vi "Publish To Topic.vi"(8 "error in (no error)":errorcluster, 9 "Message":string, 10 "Subject(\"\")":string, 11 "Topic in":refnum<class "Topic.lvclass">) -> (0 "error out":errorcluster, 3 "Topic out":refnum<class "Topic.lvclass">)   [LabVIEW 2018, in "NI_AWS_SNS.lvlib" / "Topic.lvclass"]
doc: "Publish a message to a SNS topic"
uses:
  Topic.lvclass
  C:/labview-projects/aws-toolkit/source/Core/ARN/ARN.lvclass
  C:/labview-projects/aws-toolkit/source/Core/HTTP Request/HTTP Request.lvclass
  Core/HTTP Request/Request Options.ctl
  Core/HTTP Request/Name Value Pair.ctl
  Core/HTTP Request/Region handling.ctl
  Core/HTTP Request/URL formatting.ctl
  Core/ARN/ARN.lvclass/ARN.ctl
  Core/ARN/Read ARN.vi
  Core/HTTP Request/HTTP Request.lvclass
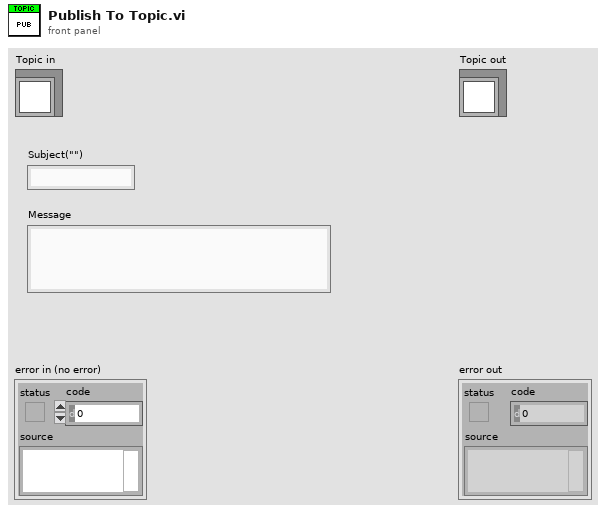
[diagram p1: front panel]
types:
  T1 = typedef "NI_AWS_Core.lvlib/HTTP Request.lvclass/Name Value Pair.ctl" = cluster{"name":string, "value":string}
  T2 = typedef "NI_AWS_Core.lvlib/HTTP Request.lvclass/Request Options.ctl" = cluster{"request headers":T1[], "request parameters":T1[], "request body":string, "region handling":T3, "URL formatting":T4}
  T3 = typedef "NI_AWS_Core.lvlib/HTTP Request.lvclass/Region handling.ctl" = enum16{"use region everywhere", "use region (authentication only)", "use region (URL only)", "ignore region everwhere"}
  T4 = typedef "NI_AWS_Core.lvlib/HTTP Request.lvclass/URL formatting.ctl" = enum16{"region-", "region."}
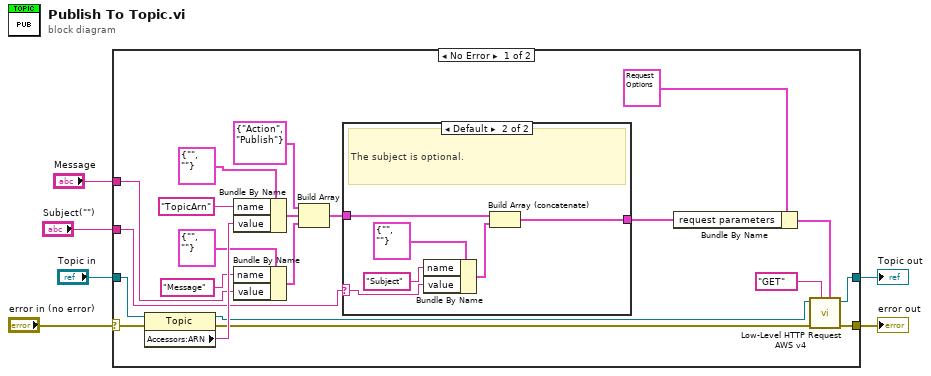
[diagram p0: block diagram]
diagram:
  n1 = case shown="No Error" "error in (no error)" {
    selector: "error in (no error)" -> [w11 w36]
    tunnel: [w14 w36] -> w5
    tunnel: [w13 w35] -> w3
    tunnel: "Topic in" -> [w15 w35]
    tunnel: "Message" -> [w12 _]
    tunnel: "Subject(\"\")" -> [w7 _]
    frame No Error {
      n2 = property class="Topic"(reference=w15, error in=w11) -> (reference out=w18:refnum<class "Topic.lvclass">, error out=w10:errorcluster, "Accessors:ARN"=w22:string)
      n3 = Bundle By Name(cluster=T1 {"name"="", "value"=""} ("Name Value Pair"), "name"="TopicArn", "value"=w22) -> (w24:T1)
      n4 = Bundle By Name(cluster=T1 {"name"="", "value"=""} ("element"), "name"="Message", "value"=w12) -> (w21:T1)
      n5 = Build Array(T1 {"name"="Action", "value"="Publish"} ("Name Value Pair"), w24, w21) -> (w9:T1[])
      n6 = case shown="Default" w7 {
        selector: w7 -> [_ w29]
        tunnel: w9 -> [w28 w34]
        tunnel: [w28 w33] -> w8
        frame "" {
          # "No subject provided. This prevents an\nerror which is thrown in caes of an\nempty string as a subject. The subject of this\nmessage will be null"
        }
        frame Default {
          # "The subject is optional."
          n7 = Bundle By Name(cluster=T1 {"name"="", "value"=""} ("element"), "name"="Subject", "value"=w29) -> (w30:T1)
          n8 = Build Array (concatenate)(w34, w30) -> (w33:T1[])
        }
      }
      n9 = Bundle By Name(cluster=T2 {"request headers"=[], "request parameters"=[], "request body"="", "region handling"=enum."use region everywhere", "URL formatting"=enum."region."} ("Request Options"), "request parameters"=w8) -> (w17:T2)
      n10 = call "Low-Level HTTP Request AWS v4.vi"("Request Options"=w17, "HTTP-Verb"="GET", "error in (no error)"=w10, "AWS Core in"=w18) -> ("error out"=w14:errorcluster, "AWS Core out"=w13:refnum<class "Topic.lvclass">)  [unwired: 4 in, 2 out]
    }
    frame Error {
    }
  }
  "error out" <- w5
  "Topic out" <- w3
